vi "Send Configure Desired Output State.vi"(7 "Message Priority (Normal)":T1=enum."Normal", 8 "error in (no error)":errorcluster, 9 "output state (Constant Voltage)":i32(ring) items=["Constant Voltage"=0, "Constant Current"=1, "Unregulated"=4, "Over Voltage"=2, "Over Current"=3], 10 "channel name (\"CHANNEL1\")":string="CHANNEL1", 11 "Message Enqueuer":refnum<class "Message Enqueuer.lvclass">) -> (0 "error out":errorcluster, 3 "Message Enqueuer out":refnum<class "Message Enqueuer.lvclass">)   [LabVIEW 2015, in "CS++DCPwr.lvlib" / "Configure Desired Output State Msg.lvclass"]
doc: "Sends the <B>CS++DCPwr.lvlib:Configure Desired Output State Msg.lvclass</B> message.\n\n<B>CS++DCPwr.lvlib:CS++DCPwr.lvclass:Configure Desired Output State.vi</B> Description:\n\nThis VI returns whether the power supply is in a particular output state.\n\nA constant voltage condition occurs when the output voltage is equal to the value of the IviDCPwr>>Basic Operation>>Voltage Level property and the current is less than or equal to the value of the IviDCPwr>>Basic Operation>>Current Limit property.\n\nA constant current condition occurs when the output current is equal to the value of the IviDCPwr>>Basic Operation>>Current Limit property and the IviDCPwr>>Basic Operation>>Current Limit Behavior property is set to IVIDCPWR_VAL_CURRENT_REGULATE.\n\nAn unregulated condition occurs when the output voltage is less than the value of the IviDCPwr>>Basic Operation>>Voltage Level property and the current is less than the value of the IviDCPwr>>Basic Operation>>Current Limit property.\n\nAn over-voltage condition occurs when the output voltage is equal to or greater than the value of the IviDCPwr>>Basic Operation>>OVP Limit property and the IviDCPwr>>Basic Operation>>OVP Enabled property is set to TRUE.\n\nAn over-current condition occurs when the output current is equal to or greater than the value of the IviDCPwr>>Basic Operation>>Current Limit property and the IviDCPwr>>Basic Operation>>Current Limit Behavior property is set to IVIDCPWR_VAL_CURRENT_TRIP. \n\nWhen either an over-voltage condition or an over-current condition occurs, the power supply's output protection disables the output. If the power supply is in an over-voltage or over-current state, it does not produce power until the output protection is reset. The IviDCPwr Reset Output Protection VI resets the output protection. Once the output protection is reset, the power supply resumes generating a power signal."
uses:
  Configure Desired Output State Msg.lvclass
  <vilib>/ActorFramework/Message Enqueuer/Message Enqueuer.lvclass
  <vilib>/ActorFramework/Message Enqueuer/Message Priority.ctl
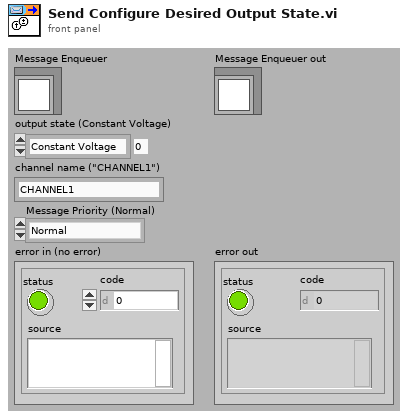
[diagram p1: front panel]
types:
  T1 = typedef "Actor Framework.lvlib/Message Enqueuer.lvclass/Message Priority.ctl" = enum16{"Low", "Normal", "High"}
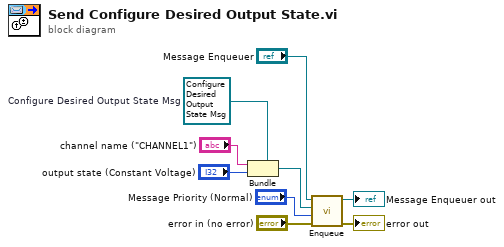
[diagram p0: block diagram]
diagram:
  w3 = refnum<class "Configure Desired Output State Msg.lvclass"> refnum  # Configure Desired Output State Msg
  n1 = Bundle(cluster=w3, "channel name (\"CHANNEL1\")", "output state (Constant Voltage)") -> (w6:refnum<class "Configure Desired Output State Msg.lvclass">)
  n2 = call <vilib>:"Enqueue.vi"("error in (no error)"="error in (no error)", "Message Priority (Normal)"="Message Priority (Normal)", "Message"=w6, "Message Enqueuer in"="Message Enqueuer") -> ("error out"=→"error out":errorcluster, "Message Enqueuer out"=→"Message Enqueuer out":refnum<class "Message Enqueuer.lvclass">)  [unwired: 6 in]
